vi "adam-read-&-parse-analog.vi"(7 "Analog Data":T1, 8 "error in (no error)":errorcluster, 9 "Bytes at Port":u32, 11 "VISA Refnum in":refnum<visa-resource-name>) -> (0 "error out":errorcluster, 1 "status  out":string, 2 "read buffer":string, 3 "VISA Refnum out":refnum<visa-resource-name>, 4 "acknowledge char":string, 5 "Analog Data Out":T1)   [LabVIEW 2020]
uses:
  controls/depreciated/analog-data-cluster.ctl
panel:
  out "read return":u32
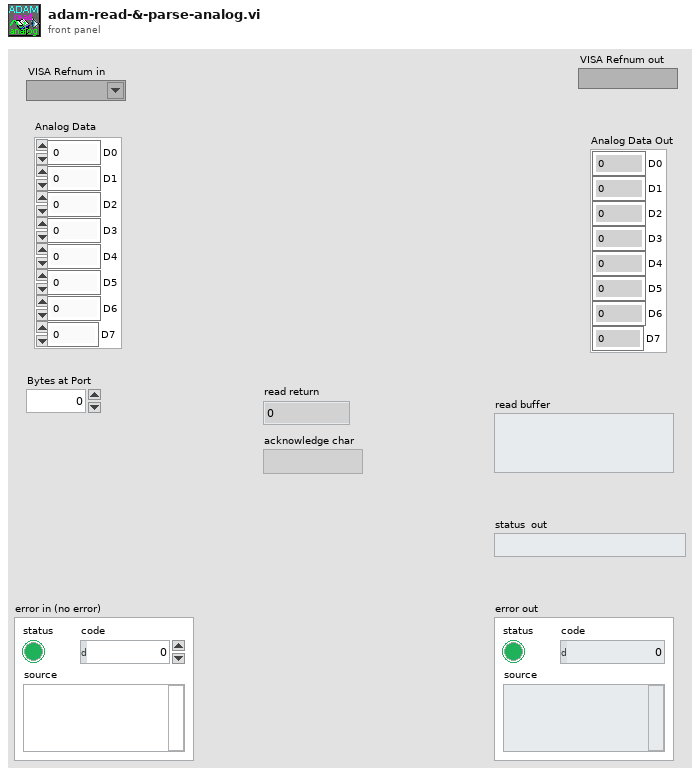
[diagram p1: front panel]
types:
  T1 = typedef "analog-data-cluster.ctl" = cluster{"D0":dbl, "D1":dbl, "D2":dbl, "D3":dbl, "D4":dbl, "D5":dbl, "D6":dbl, "D7":dbl}
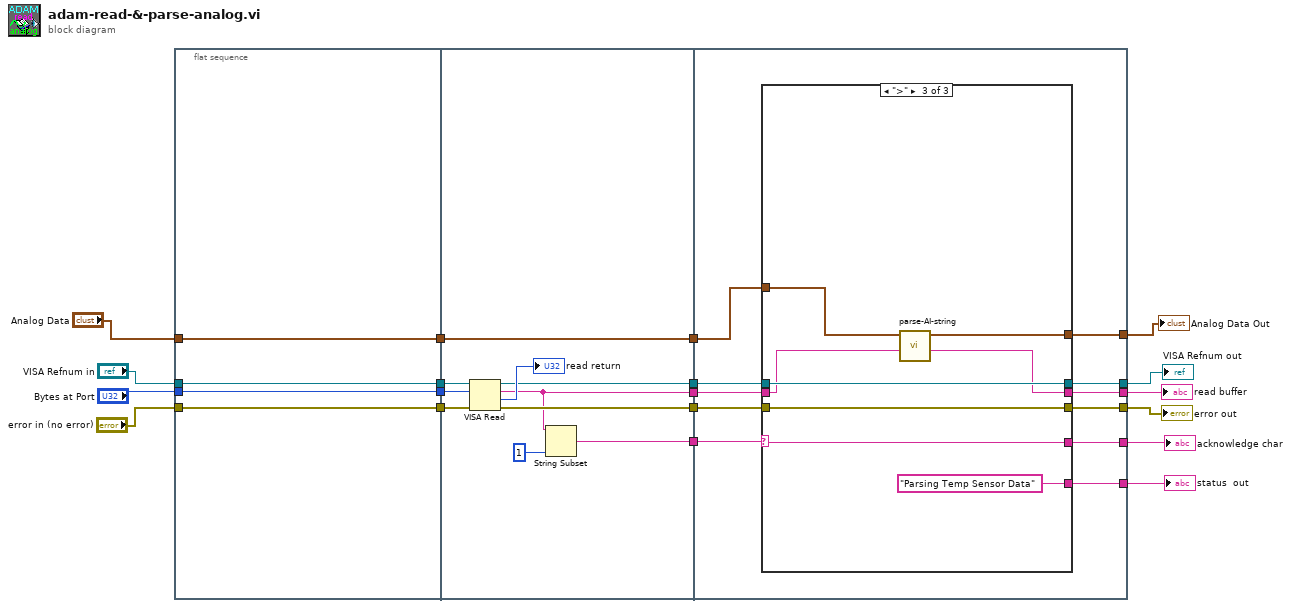
[diagram p0: block diagram]
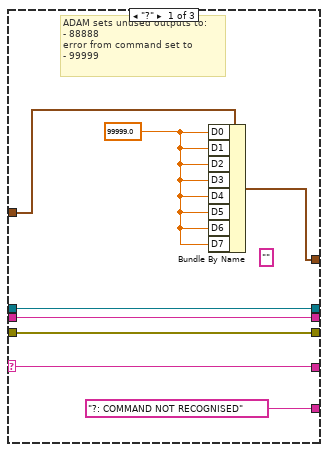
[diagram p2: hidden frame]
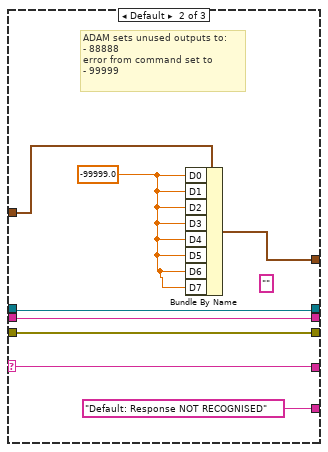
[diagram p3: hidden frame]
diagram:
  n1 = flat-sequence {
    tunnel: [w23] -> w19
    tunnel: "VISA Refnum in" -> [w23]
    tunnel: [w22] -> w17
    tunnel: "Bytes at Port" -> [w22]
    tunnel: [w21] -> w15
    tunnel: "error in (no error)" -> [w21]
    tunnel: [w20] -> w13
    tunnel: "Analog Data" -> [w20]
    tunnel: w19 -> [w27]
    tunnel: w17 -> [w26]
    tunnel: w15 -> [w25]
    tunnel: w13 -> [w24]
    tunnel: [w31] -> w12
    tunnel: [w30] -> w11
    tunnel: [w29] -> w10
    tunnel: [w28] -> w9
    tunnel: [w24] -> w8
    tunnel: w12 -> [w35]
    tunnel: w11 -> [w36]
    tunnel: w10 -> [w43]
    tunnel: w9 -> [w44]
    tunnel: w8 -> [w42]
    tunnel: [w41] -> w7
    tunnel: [w40] -> w6
    tunnel: [w39] -> w5
    tunnel: [w38] -> w4
    tunnel: [w37] -> w3
    tunnel: [w34] -> w2
    frame #0 {
    }
    frame #1 {
      n2 = VISA Read(VISA resource name=w27, byte count=w26, error in (no error)=w25) -> (VISA resource name out=w28:refnum<visa-resource-name>, read buffer=w29:string, return count=→"read return":u32, error out=w30:errorcluster)
      n3 = String Subset(string=w29, length (rest)=1 ("length (rest)")) -> (substring=w31:string)  [unwired: 1 in]
    }
    frame #2 {
      n4 = case shown="\">\"" w35 {
        selector: w35 -> [w46 w54 w65]
        tunnel: [w51 w59 w61] -> w41
        tunnel: [w52 w60 w67] -> w40
        tunnel: [w50 w58 w66] -> w39
        tunnel: [w48 w55 w62] -> w38
        tunnel: ["?: COMMAND NOT RECOGNISED" ("status") "Default: Response NOT RECOGNISED" ("status") "Parsing Temp Sensor Data" ("status")] -> w37
        tunnel: w44 -> [w52 w60 w67]
        tunnel: w36 -> [w50 w58 w66]
        tunnel: w43 -> [w51 w59 w63]
        tunnel: w42 -> [w47 w56 w64]
        tunnel: [w46 w54 w65] -> w34
        frame "?" {
          w45 = 99999.0 ("T1")
          (unwired) "" ("csv")
          # "ADAM sets unused outputs to:\n- 88888\nerror from command set to\n- 99999"
          n5 = Bundle By Name(cluster=w47, "D0"=w45, "D1"=w45, "D2"=w45, "D3"=w45, "D4"=w45, "D5"=w45, "D6"=w45, "D7"=w45) -> (w48:T1)
        }
        frame Default {
          w53 = -99999.0 ("T1")
          (unwired) "" ("csv")
          # "ADAM sets unused outputs to:\n- 88888\nerror from command set to\n- 99999"
          n6 = Bundle By Name(cluster=w56, "D0"=w53, "D1"=w53, "D2"=w53, "D3"=w53, "D4"=w53, "D5"=w53, "D6"=w53, "D7"=w53) -> (w55:T1)
        }
        frame ">" {
          n7 = call "parse-AI-string.vi"("read buffer in"=w63, "Analog Data"=w64) -> ("csv"=w61:string, "Analog Data Out"=w62:T1)  [unwired: 8 in]
        }
      }
    }
  }
  "status  out" <- w3
  "VISA Refnum out" <- w6
  "read buffer" <- w7
  "error out" <- w5
  "acknowledge char" <- w2
  "Analog Data Out" <- w4
